vi "读取当前抽取数据数组.vi"(8 "error in (no error)":errorcluster caption="错误输入（无错误）", 11 "抽取参数输入":refnum<class "抽取参数.lvclass">) -> (0 "error out":errorcluster caption="错误输出", 2 "当前抽取数据数组":string[](array[string]), 3 "抽取参数输出":refnum<class "抽取参数.lvclass">)   [LabVIEW 2020, in "抽取参数.lvclass"]
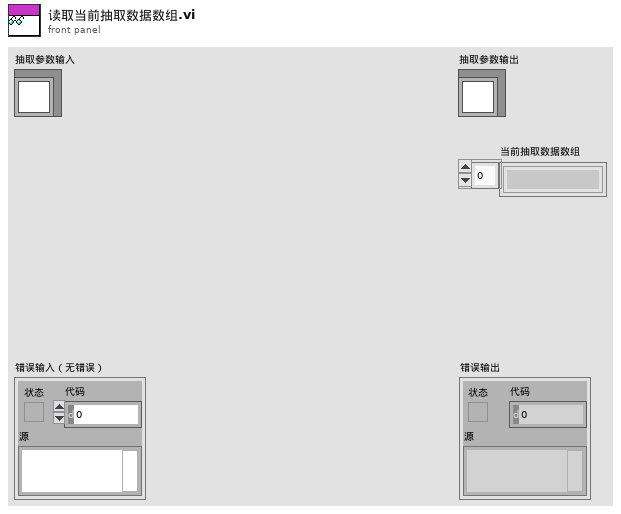
[diagram p1: front panel]
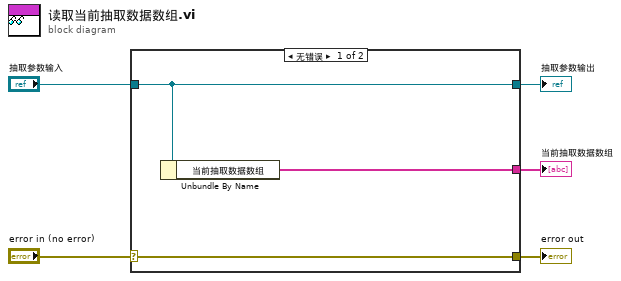
[diagram p0: block diagram]
diagram:
  n1 = case shown="无错误" "error in (no error)" {
    selector: "error in (no error)" -> [w8 w9]
    tunnel: [w8 w9] -> w4
    tunnel: [w7 w10] -> w2
    tunnel: "抽取参数输入" -> [w7 w10]
    tunnel: [w6 _] -> w1
    frame No Error {
      n2 = Unbundle By Name(w7) -> ("当前抽取数据数组"=w6:string[])
    }
    frame Error {
    }
  }
  "error out" <- w4
  "抽取参数输出" <- w2
  "当前抽取数据数组" <- w1
